vi "LATITUD-LONGITUD.vi"(2 "DIRECCION LONGITUD":string, 3 "VALOR LONGITUD":string, 4 "DIRECCION LATITUD":string, 5 "VALOR  LATITUD":string) -> (0 "LONGITUD":string, 1 "LATITUD":string)   [LabVIEW 2020]
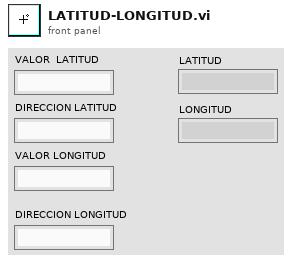
[diagram p1: front panel]
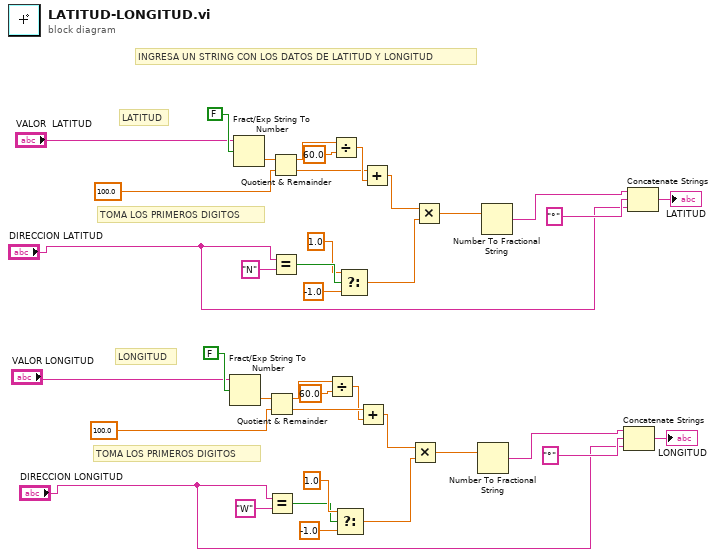
[diagram p0: block diagram]
diagram:
  # "TOMA LOS PRIMEROS DIGITOS"
  # "LONGITUD"
  # "TOMA LOS PRIMEROS DIGITOS"
  # "LATITUD"
  # "INGRESA UN STRING CON LOS DATOS DE LATITUD Y LONGITUD"
  n1 = Fract/Exp String To Number(use system decimal point (T)=FALSE, string="VALOR LONGITUD") -> (number=w11:dbl)  [unwired: 2 in, 1 out]
  n2 = Fract/Exp String To Number(use system decimal point (T)=FALSE, string="VALOR  LATITUD") -> (number=w32:dbl)  [unwired: 2 in, 1 out]
  n3 = Quotient & Remainder(x=w11, y=100.0) -> (x-y*floor(x/y)=w6:dbl, floor(x/y)=w9:dbl)
  n4 = Equal?(x="DIRECCION LONGITUD", y="W") -> (x = y?=w13:bool)
  n5 = Quotient & Remainder(x=w32, y=100.0) -> (x-y*floor(x/y)=w37:dbl, floor(x/y)=w34:dbl)
  n6 = Equal?(x="DIRECCION LATITUD", y="N") -> (x = y?=w30:bool)
  n7 = Divide(x=w6, y=60.0) -> (x/y=w8:dbl)
  n8 = Divide(x=w37, y=60.0) -> (x/y=w35:dbl)
  n9 = Select(t=1.0, s=w13, f=-1.0) -> (s? t:f=w16:dbl)
  n10 = Select(t=1.0, s=w30, f=-1.0) -> (s? t:f=w27:dbl)
  n11 = Add(x=w9, y=w8) -> (x+y=w15:dbl)
  n12 = Add(x=w34, y=w35) -> (x+y=w28:dbl)
  n13 = Multiply(x=w15, y=w16) -> (x*y=w14:dbl)
  n14 = Multiply(x=w28, y=w27) -> (x*y=w29:dbl)
  n15 = Number To Fractional String(number=w14) -> (F-format string=w19:string)  [unwired: 3 in]
  n16 = Number To Fractional String(number=w29) -> (F-format string=w24:string)  [unwired: 3 in]
  n17 = Concatenate Strings(w19, "°", "DIRECCION LONGITUD") -> (→"LONGITUD":string)
  n18 = Concatenate Strings(w24, "°", "DIRECCION LATITUD") -> (→"LATITUD":string)
